vi "Register LabVIEW QObject.vi"(5 "Direct Ancestor (Type Only)":refnum<class "LQObject.lvclass">, 8 "Error In":errorcluster, 10 "New Signals":string[](array[string]), 11 "Custom LQObject In":refnum<class "LQObject.lvclass">) -> (0 "Error Out":errorcluster, 3 "Custom LQObject Out":refnum<class "LQObject.lvclass">)   [LabVIEW 2014, in "LQ Core.lvlib" / "LQObject.lvclass"]
uses:
  LQObject.lvclass
  LQIdentity/LQIdentity.lvclass/LQIdentity.ctl
  LQIdentity/LQIdentity.lvclass
  LQ Core.lvlib
panel:
  # "Copyright (c) 2016 Sze Howe Koh\n\nThis Source Code Form is subject to the terms of the Mozilla Public\nLicense, v. 2.0. If a copy of the MPL was not distributed with this\nfile, You can obtain one at http://mozilla.org/MPL/2.0/."
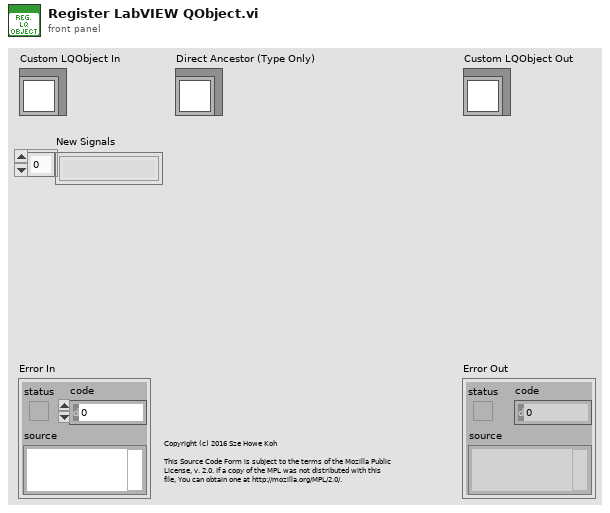
[diagram p1: front panel]
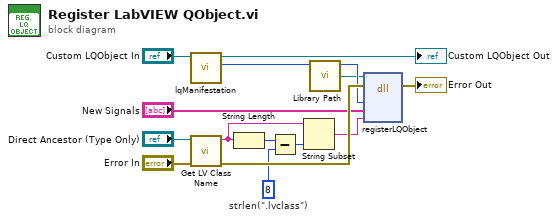
[diagram p0: block diagram]
diagram:
  w8 = 8  # strlen(".lvclass")
  n1 = call "lqManifestation.vi"("LQIdentity in"="Custom LQObject In") -> ("Manifestation"=w10:u64, "LQIdentity out"=→"Custom LQObject Out":refnum<class "LQObject.lvclass">)  [unwired: 9 in]
  n2 = call <vilib>:"Get LV Class Name.vi"("error in (no error)"="Error In", "object"="Direct Ancestor (Type Only)") -> ("error out"=w14:errorcluster, "class name"=w6:string)  [unwired: 8 in]
  n3 = String Length(string=w6) -> (length=w9:i32)
  n4 = Subtract(x=w9, y=w8) -> (x-y=w7:i32)
  n5 = String Subset(string=w6, length (rest)=w7) -> (substring=w3:string)  [unwired: 1 in]
  n6 = call "Library Path.vi"() -> ("Library Path"=w1:path)
  n7 = dll-call lib="?" fn="registerLQObject"(path in=w1, error in=w14, "_instance"=w10, "signalList"="New Signals", "superClassName"=w3) -> (error out=→"Error Out":errorcluster)  [unwired: 5 in, 1 out]
